vi "echo.vi"(8 "error in (no error)":errorcluster, 11 "params":refnum<class "JSON Value.lvclass">) -> (0 "error out":errorcluster, 3 "data":refnum<class "JSON Value.lvclass">)   [LabVIEW 2017]
uses:
  <vilib>/NI/JSON Support for LabVIEW/JSON Value/JSON Value.lvclass
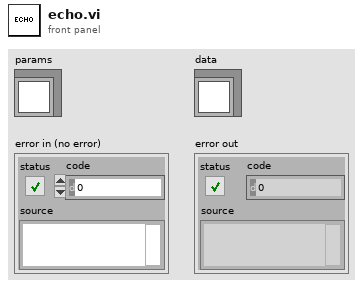
[diagram p1: front panel]
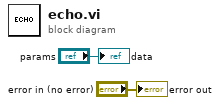
[diagram p0: block diagram]
diagram:
  "data" <- "params"
  "error out" <- "error in (no error)"
